vi "Configure User-Defined Codes.vi"(8 "Error In":errorcluster, 11 "User-Defined Codes":i32[](array[numeric])) -> (0 "Error Out":errorcluster)   [LabVIEW 2025, in "LOGlib_LV2025.lvlib"]
doc: "Adds user-defined error codes to the logging statement so user errors are properly formatted into Comma-Separated Values (CSV) lines."
uses:
  LOGlib_LV2025.lvlib
  Support/Error/Action.ctl
  Support/Error/Error.lvlib
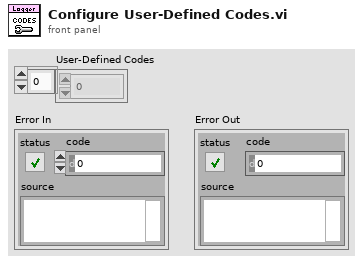
[diagram p1: front panel]
types:
  T1 = typedef "LOGlib_LV2025.lvlib/Error.lvlib/Action.ctl" = enum16{"Initialize", "Get", "Set Verbosity", "Set User-Defined Codes", "Set User-Defined Descriptions", "Shutdown"}
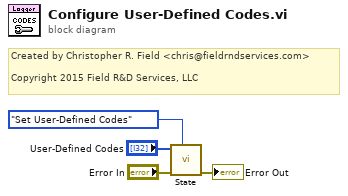
[diagram p0: block diagram]
diagram:
  # "Created by Christopher R. Field <chris@fieldrndservices.com>\n\nCopyright 2015 Field R&D Services, LLC"
  n1 = call "State.vi"("Action"=Action."Set User-Defined Codes", "Error In"="Error In", "Set Value"="User-Defined Codes") -> ("Error Out"=→"Error Out":errorcluster)  [unwired: 7 in, 1 out]
